vi "niDTS WLAN Dut Tx Abort.vi"(0 "WLAN Dut Handle in":T1, 11 "error in (no error)":errorcluster) -> (4 "WLAN Dut Handle out":T1, 15 "error out":errorcluster)   [LabVIEW 2015, in "niDTS WLAN.lvlib"]
uses:
  niDTS WLAN.lvlib
  Framework/Dut/Includes/niDTS Dut INC Handle.ctl
  Framework/Dut/Objects/BASE_class/niDTS Dut.lvclass
  Includes/niDTS WLAN Dut INC Handle.ctl
  Objects/BASE_class/niDTS WLAN Dut.lvclass
  Framework/niDTS Framework.lvlib
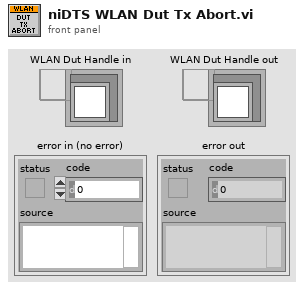
[diagram p1: front panel]
types:
  T1 = typedef "niDTS Framework.lvlib/niDTS Dut INC Handle.ctl" = refnum<data-value>
  T2 = typedef "niDTS WLAN.lvlib/niDTS WLAN Dut INC Handle.ctl" = refnum<data-value>
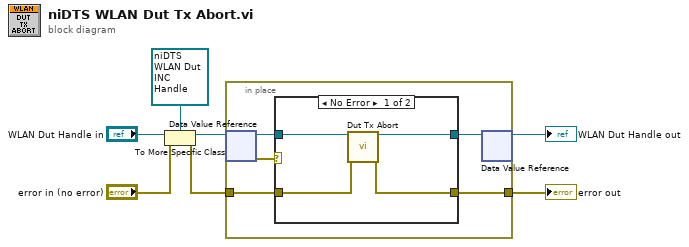
[diagram p0: block diagram]
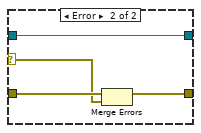
[diagram p2: hidden frame]
diagram:
  n1 = To More Specific Class(target class=T2 refnum ("WLAN Dut Handle in"), reference="WLAN Dut Handle in", error in="error in (no error)") -> (specific class reference=w4:T2, error out=w1:errorcluster)
  n2 = in-place {
    in-place-border: w1 -> [w9]
    in-place-border: [w8] -> w5
    n3 = in-place-dvr #1(w4) -> (w11:refnum<class "niDTS WLAN Dut.lvclass">, w12:errorcluster)
    n4 = case shown="No Error" w12 {
      selector: w12 -> [_ w18]
      tunnel: w11 -> [w16 w20]
      tunnel: [w13 w20] -> w10
      tunnel: w9 -> [w15 w19]
      tunnel: [w14 w17] -> w8
      frame No Error {
        n5 = call-dynamic "Dut Tx Abort.vi"("niDTS DUT in"=w16, "error in (no error)"=w15) -> ("niDTS DUT out"=w13:refnum<class "niDTS WLAN Dut.lvclass">, "error out"=w14:errorcluster)  [unwired: 12 in]
      }
      frame Error {
        n6 = Merge Errors(w19, w18) -> (w17:errorcluster)
      }
    }
    n7 = in-place-dvr #1(w10) -> (→"WLAN Dut Handle out":T2)  [unwired: 1 out]
  }
  "error out" <- w5
